vi "ExamplePicRing.vi"() -> ()   [LabVIEW 2017]
uses:
  20898ad1-9fc1-493d-921a-c5c61ee88547.vi
  8a370903-fa1a-41ba-a2f2-fd9372dfcc71.vi
panel:
  in  "Ring":u16(ring)
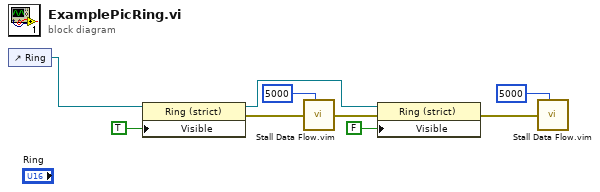
[diagram p0: block diagram]
diagram:
  n1 = control-ref of="Ring"() -> (w1:refnum<vi>)
  n2 = property class="Ring (strict)"(reference=w1, "Visible"=TRUE) -> (reference out=w6:refnum<vi>, error out=w8:errorcluster)  [unwired: 1 in]
  n3 = call "Stall Data Flow.vim"("value in"=w8, "milliseconds to wait"=u32 5000) -> ("value out"=w7:errorcluster)  [unwired: 1 out]
  n4 = property class="Ring (strict)"(reference=w6, error in=w7, "Visible"=FALSE) -> (error out=w3:errorcluster)  [unwired: 1 out]
  n5 = call "Stall Data Flow.vim"("value in"=w3, "milliseconds to wait"=u32 5000) -> ()  [unwired: 2 out]
